vi "Array from start-stop-step.vi"(1 "Step":dbl, 2 "Stop":dbl, 3 "Start":dbl) -> (0 "Array of numbers":dbl[](array[numeric]))   [LabVIEW 2009, in "Varian Magnet.lvclass"]
uses:
  Varian Magnet.lvclass
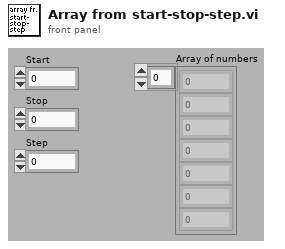
[diagram p1: front panel]
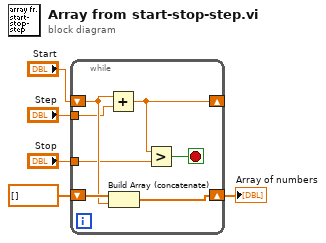
[diagram p0: block diagram]
diagram:
  n1 = while {
    shift-right: [w11] -> w5
    shift-left: dbl[] [] -> [w12]
    shift-right: [w9] -> _
    shift-left: "Start" -> [w10]
    tunnel: "Stop" -> [w7]
    tunnel: "Step" -> [w6]
    stop <- w8 stop-if-true
    n2 = Add(x=w10, y=w6) -> (x+y=w9:dbl)
    n3 = Build Array (concatenate)(w12, w10) -> (w11:dbl[])
    n4 = Greater?(x=w9, y=w7) -> (0:w8:bool)
  }
  "Array of numbers" <- w5
